vi "go_to_BBO_position.vi"(0 "Set BBO crystal position":i32, 11 "error in (no error)":errorcluster) -> (4 "BBO crystal position":i32, 13 "Sucessful?":bool, 15 "error out":errorcluster)   [LabVIEW 2023]
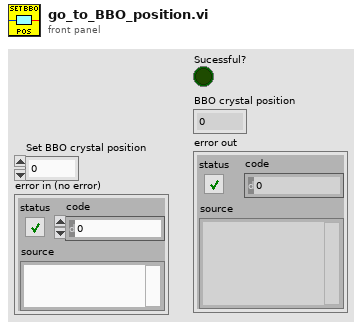
[diagram p1: front panel]
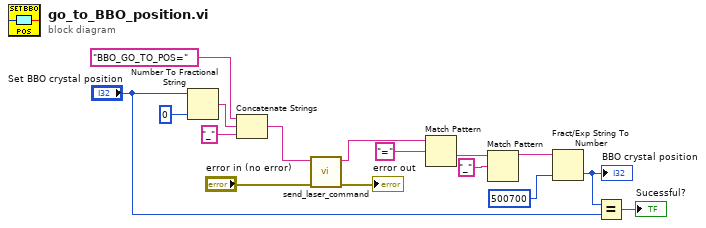
[diagram p0: block diagram]
diagram:
  n1 = Number To Fractional String(number="Set BBO crystal position", precision (6)=i16 0) -> (F-format string=w7:string)  [unwired: 2 in]
  n2 = Concatenate Strings("BBO_GO_TO_POS=", w7, "_" ("string")) -> (w5:string)
  n3 = call "send_laser_command.vi"("error in (no error)"="error in (no error)", "String"=w5) -> ("error out"=→"error out":errorcluster, "data out"=w10:string)  [unwired: 8 in]
  n4 = Match Pattern(string=w10, regular expression="=") -> (after substring=w13:string)  [unwired: 1 in, 3 out]
  n5 = Match Pattern(string=w13, regular expression="_") -> (before substring=w11:string)  [unwired: 1 in, 3 out]
  n6 = Fract/Exp String To Number(string=w11, default (0 dbl)=500700 ("Set BBO crystal position")) -> (number=w2:i32)  [unwired: 2 in, 1 out]
  "BBO crystal position" <- w2
  n7 = Equal?(x=w2, y="Set BBO crystal position") -> (x = y?=→"Sucessful?":bool)
